vi "Peak_Base_Error_Check (SubVI).vi"(9 "Model Flow":waveform(dbl), 10 "T_Ejection Period (s)":dbl, 11 "T_Flow Peak (s)":dbl) -> (0 "T Base":dbl, 1 "T Peak":dbl, 2 "Error":dbl[](array[numeric]), 3 "Logic":bool)   [LabVIEW 2017]
panel:
  out "x-y":dbl
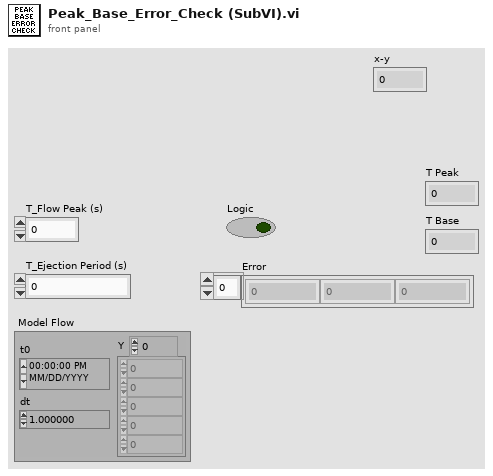
[diagram p1: front panel]
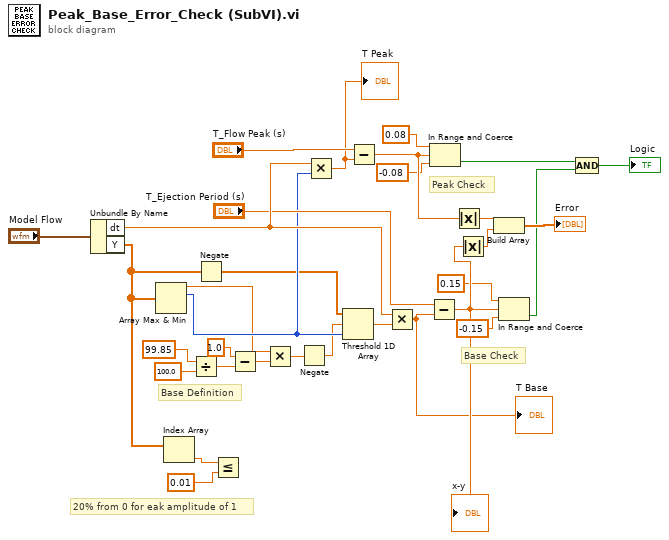
[diagram p0: block diagram]
diagram:
  # "20% from 0 for eak amplitude of 1"
  # "Base Check"
  # "Peak Check"
  # "Base Definition"
  n1 = Unbundle By Name("Model Flow") -> ("dt"=w28:dbl, "Y"=w6:dbl[])
  n2 = Array Max & Min(array=w6) -> (max value=w13:dbl, max index (indices)=w22:i32)  [unwired: 2 out]
  n3 = Index Array(array=w6) -> (element=w5:dbl)  [unwired: 1 in]
  n4 = Divide(x=99.85 ("Numeric"), y=100.0 ("start")) -> (x/y=w8:dbl)
  n5 = Negate(x=w6) -> (-x=w16:dbl[])
  n6 = Less Or Equal?(x=w5, y=0.01 ("Numeric")) -> ()  [unwired: 1 out]
  n7 = Subtract(x=1.0 ("start"), y=w8) -> (x-y=w12:dbl)
  n8 = Multiply(x=w13, y=w12) -> (x*y=w14:dbl)
  n9 = Negate(x=w14) -> (-x=w15:dbl)
  n10 = Multiply(x=w28, y=w22) -> (x*y=w21:dbl)
  "T Peak" <- w21
  n11 = Threshold 1D Array(1:w22, 2:w15, 3:w16) -> (0:w17:dbl)
  n12 = Subtract(x="T_Flow Peak (s)", y=w21) -> (x-y=w30:dbl)
  n13 = Multiply(x=w28, y=w17) -> (x*y=w18:dbl)
  "T Base" <- w18
  n14 = Subtract(x="T_Ejection Period (s)", y=w18) -> (x-y=w32:dbl)
  "x-y" <- w32
  n15 = In Range and Coerce(upper limit=0.08, x=w30, lower limit=-0.08) -> (In Range?=w3:bool)  [unwired: 1 out]
  n16 = Absolute Value(x=w30) -> (abs(x)=w29:dbl)
  n17 = Absolute Value(x=w32) -> (abs(x)=w31:dbl)
  n18 = Build Array(w29, w31) -> (→"Error":dbl[])
  n19 = In Range and Coerce(upper limit=0.15, x=w32, lower limit=-0.15) -> (In Range?=w2:bool)  [unwired: 1 out]
  n20 = Compound Arithmetic op=AND(w3, w2) -> (→"Logic":bool)
